vi "Main_function.vi"() -> ()   [LabVIEW 2014]
uses:
  <vilib>/DAQmx/write.llb/DAQmx Write (Analog DBL 1Chan 1Samp).vi
  <vilib>/DAQmx/write.llb/DAQmx Write (Analog 1D DBL NChan 1Samp).vi
  <vilib>/DAQmx/read.llb/DAQmx Read (Analog 1D Wfm NChan NSamp).vi
panel:
  out "Waveform Chart":waveform(dbl)(graph)
  out "?":waveform(dbl)
  in  "Boolean 2":bool
  out "Encoder":dbl format="%#_13g"
  out "?":waveform(dbl)
  out "Torque Transducer":dbl=-0.04652723592105682 format="%#.3g"
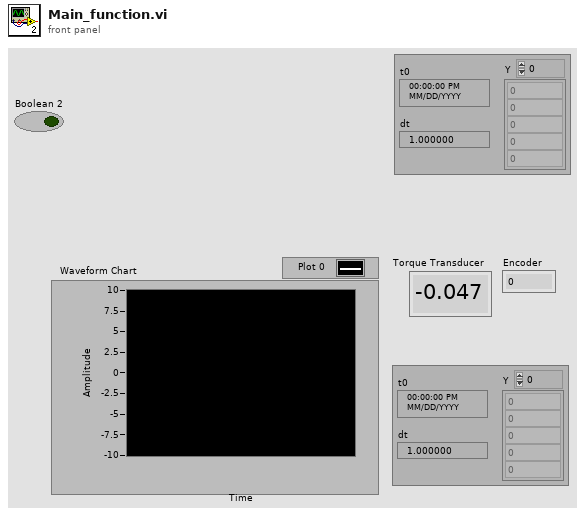
[diagram p1: front panel]
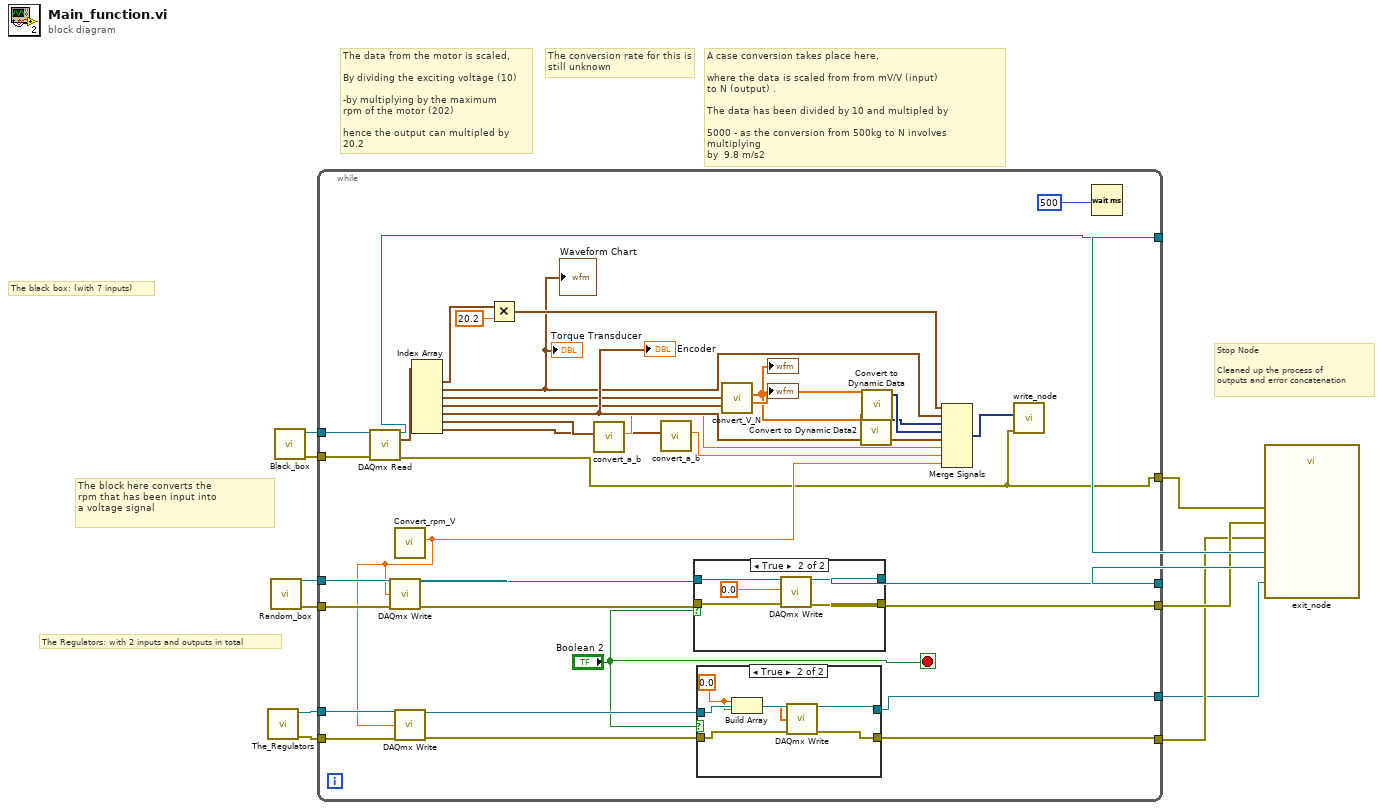
[diagram p0: block diagram]
diagram:
  # "The Regulators: with 2 inputs and outputs in total"
  # "The black box: (with 7 inputs)"
  # "Stop Node\n\nCleaned up the process of\noutputs and error concatenation"
  # "The conversion rate for this is \nstill unknown"
  # "The block here converts the \nrpm that has been input into \na voltage signal"
  # "A case conversion takes place here, \n\nwhere the data is scaled from from mV/V (input) \nto N (output) . \n\nThe data has been divided by 10 and multipled by\n\n5000 - as the conversion from 500kg to N involves multiplying \nby  9.8 m/s2"
  # "The data from the motor is scaled,\n\nBy dividing the exciting voltage (10) \n\n-by multiplying by the maximum \nrpm of the motor (202)  \n\nhence the output can multipled by 20.2"
  n1 = call "The_Regulators.vi"() -> ("Error Out"=w7:errorcluster, "DAQmx Task Name"=w8:refnum<k21>)  [unwired: 10 in]
  n2 = call "Random_box.vi"() -> ("Error Out"=w9:errorcluster, "Task Out"=w10:refnum<k21>)  [unwired: 10 in]
  n3 = call "Black_box.vi"() -> ("error out"=w11:errorcluster, "task out"=w12:refnum<k21>)  [unwired: 10 in]
  n4 = while {
    tunnel: w12 -> [w48]
    tunnel: w11 -> [w47]
    tunnel: w10 -> [w41]
    tunnel: w9 -> [w40]
    tunnel: w8 -> [w37]
    tunnel: w7 -> [w36]
    tunnel: [w33] -> w1
    tunnel: [w32] -> w2
    tunnel: [w30] -> w4
    tunnel: [w31] -> w3
    tunnel: [w16] -> w5
    tunnel: [w13] -> w6
    stop <- "Boolean 2" stop-if-true
    n5 = call-poly <vilib>:"DAQmx Read.vi"("task/channels in"=w48, "error in"=w47) -> ("task out"=w16:refnum<k21>, "data"=w46:waveform(dbl)[], "error out"=w13:errorcluster)  [unwired: 11 in]
    n6 = call "Convert_rpm_V.vi"() -> (2:w23:dbl)  [unwired: 11 in]
    n7 = call-poly <vilib>:"DAQmx Write.vi"("task/channels in"=w41, "data"=w23, "error in"=w40) -> ("task out"=w39:refnum<k21>, "error out"=w38:errorcluster)  [unwired: 10 in, 1 out]
    n8 = call-poly <vilib>:"DAQmx Write.vi"("task/channels in"=w37, "data"=w23, "error in"=w36) -> ("task out"=w35:refnum<k21>, "error out"=w34:errorcluster)  [unwired: 10 in, 1 out]
    n9 = Index Array(array=w46) -> (element #1=w43:waveform(dbl), element #2=w15:waveform(dbl), element #3=w22:waveform(dbl), element #4=w21:waveform(dbl), element #5=w42:waveform(dbl), element #6=w29:waveform(dbl), element #7=w26:waveform(dbl))  [unwired: 7 in]
    "Torque Transducer" <- w15
    "Encoder" <- w42
    "Waveform Chart" <- w15
    n10 = Multiply(x=w43, y=20.2) -> (x*y=w44:waveform(dbl))
    n11 = call "convert_a_b.vi"("Numeric Arrays"=w29) -> ("Output"=w28:dbl)  [unwired: 10 in]
    n12 = call "convert_a_b.vi"("Numeric Arrays"=w26) -> ("Output"=w27:dbl)  [unwired: 10 in]
    n13 = case shown="True" "Boolean 2" {
      tunnel: w39 -> [w58 w63]
      tunnel: w38 -> [w57 w62]
      tunnel: [w58 w61] -> w30
      tunnel: [w57 w60] -> w31
      frame False {
      }
      frame True {
        n14 = call-poly <vilib>:"DAQmx Write.vi"("task/channels in"=w63, "data"=0.0, "error in"=w62) -> ("task out"=w61:refnum<k21>, "error out"=w60:errorcluster)  [unwired: 10 in, 1 out]
      }
    }
    n15 = case shown="True" "Boolean 2" {
      tunnel: w35 -> [w50 w56]
      tunnel: w34 -> [w49 w55]
      tunnel: [w49 w54] -> w32
      tunnel: [w50 w53] -> w33
      frame False {
      }
      frame True {
        w52 = 0.0
        n16 = Build Array(w52, w52) -> (w51:dbl[])
        n17 = call-poly <vilib>:"DAQmx Write.vi"("task/channels in"=w56, "data"=w51, "error in"=w55) -> ("task out"=w53:refnum<k21>, "error out"=w54:errorcluster)  [unwired: 10 in, 1 out]
      }
    }
    n18 = call "convert_V_N.vi"("waveform"=w21, "waveform 2"=w22) -> ("Array"=w19:dbl[], "Array 2"=w17:dbl[])  [unwired: 8 in]
    "?" <- w19
    "?" <- w17
    n19 = call "Convert to Dynamic Data2"("Array"=w17) -> ("Dynamic Data Type"=w18:dynamicdata)  [unwired: 3 in]
    n20 = call "Convert to Dynamic Data"("Array"=w19) -> ("Dynamic Data Type"=w20:dynamicdata)  [unwired: 3 in]
    n21 = Merge Signals(w44, w15, w18, w20, w42, w28, w27, w23) -> (w14:dynamicdata)
    n22 = call "write_node.vi"("error in (no error)"=w13, "Signals"=w14) -> ()  [unwired: 9 in, 1 out]
    n23 = Wait (ms)(milliseconds to wait=u32 500 ("millisecond timer value")) -> ()  [unwired: 1 out]
  }
  n24 = call "exit_node.vi"("error in 3"=w2, "task/channels in 3"=w1, "error in 2"=w3, "task/channels in 2"=w4, "error in"=w6, "task/channels in"=w5) -> ()  [unwired: 6 in]
